vi "Generate Large Output.vi"   [LabVIEW 2024, in "Integration Tests.lvlib"]
uses:
  Integration Tests.lvlib
  CLI Class/CLI.lvclass
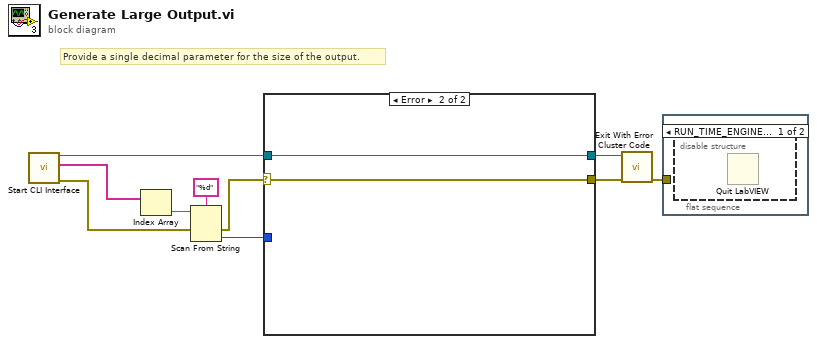
[diagram p0: block diagram]
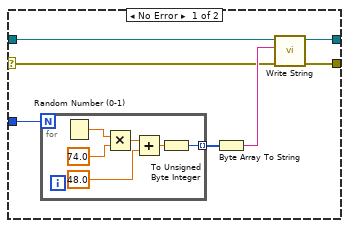
[diagram p2: hidden frame]
diagram:
  # "Provide a single decimal parameter for the size of the output."
  n1 = call "Start CLI Interface.vi"() -> ("error out"=w7:errorcluster, "Custom Parameters"=w9:string[], "CLI out"=w2:refnum<class "CLI.lvclass">)  [unwired: 8 in, 1 out]
  n2 = Index Array(array=w9) -> (element=w8:string)  [unwired: 1 in]
  n3 = Scan From String(format string="%d", input string=w8, error in=w7) -> (error out=w1:errorcluster, output 1=w5:i32)  [unwired: 2 in, 2 out]
  n4 = case shown="Error" w1 {
    selector: w1 -> [w11 w24]
    tunnel: w5 -> [w17 _]
    tunnel: [w15 w24] -> w4
    tunnel: [w14 w25] -> w3
    tunnel: w2 -> [w13 w25]
    frame No Error {
      n5 = for {
        N: w17 -> [_]
        tunnel: [w18] -> w16 mode=indexing
        n6 = Random Number (0-1)() -> (number: 0 to 1=w19:dbl)
        n7 = Multiply(x=w19, y=74.0) -> (x*y=w21:dbl)
        n8 = Add(x=w21, y=48.0) -> (x+y=w23:dbl)
        n9 = To Unsigned Byte Integer(number=w23) -> (unsigned 8bit integer=w18:u8)
      }
      n10 = Byte Array To String(unsigned byte array=w16) -> (string=w12:string)
      n11 = call "Write String.vi"("error in (no error)"=w11, "Text to Write"=w12, "CLI in"=w13) -> ("error out"=w15:errorcluster, "CLI out"=w14:refnum<class "CLI.lvclass">)  [unwired: 7 in]
    }
    frame Error {
    }
  }
  n12 = call "Exit With Error Cluster Code.vi"("error in (no error)"=w4, "CLI in"=w3) -> ("error out"=w10:errorcluster)  [unwired: 9 in]
  n13 = flat-sequence {
    tunnel: w10 -> [_]
    frame #0 {
      n14 = disable-structure shown="RUN_TIME_ENGINE==True" {
        frame condition #0 {
          n15 = Quit LabVIEW() -> ()  [unwired: 1 in]
        }
        frame condition #1 (active) {
        }
      }
    }
  }
